vi "hydrolysis_reactor_run_parallel.vi"(10 "Spec files":path[](array[path]), 11 "instances":i32) -> (2 "paths out":path[](array[path]))   [LabVIEW 2019]
uses:
  <vilib>/Utility/sysdir.llb/System Directory Type.ctl
  lib/libSimulationControl/libSimulationControl.lvlib
panel:
  # "*******************************************************************\nBiogas Plant Control\n\nAuthor: Paul Zügel\nGCSC-Frankfurt am Main 2020\n\n*******************************************************************"
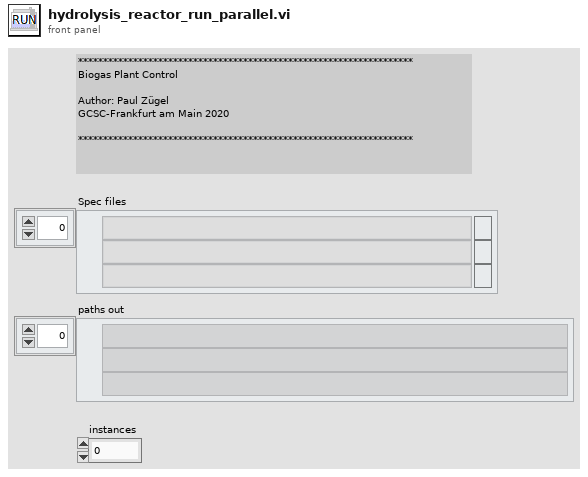
[diagram p1: front panel]
types:
  T1 = typedef "System Directory Type.ctl" = i32
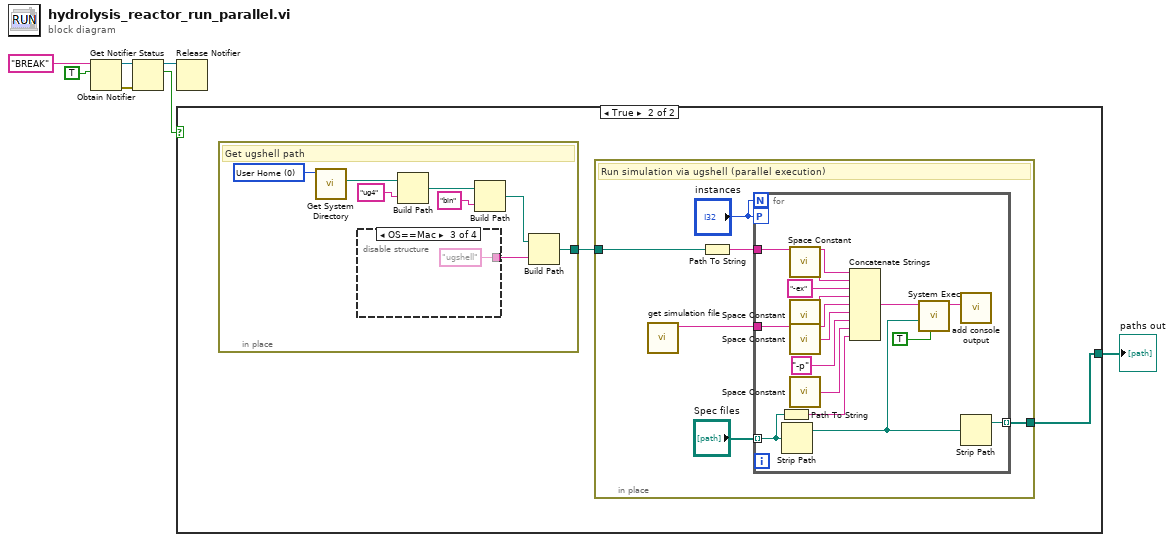
[diagram p0: block diagram]
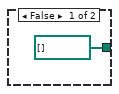
[diagram p2: hidden frame]
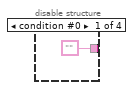
[diagram p3: hidden frame]
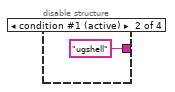
[diagram p4: hidden frame]
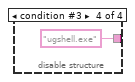
[diagram p5: hidden frame]
diagram:
  n1 = Obtain Notifier(name (unnamed)="BREAK", notification data type=TRUE) -> (notifier out=w5:refnum<notifier>, error out=w4:errorcluster)  [unwired: 2 in, 1 out]
  n2 = Get Notifier Status(notifier=w5, error in (no error)=w4) -> (notifier out=w1:refnum<notifier>, current notification=w3:bool)  [unwired: 3 out]
  n3 = Release Notifier(notifier=w1) -> ()  [unwired: 2 in, 3 out]
  n4 = case shown="True" w3 {
    tunnel: [path[] [] ("Spec files") w10] -> w2
    frame False {
    }
    frame True {
      # "Define current paths"
      # "True only on first Iteration (current_time = starttime)\nWe get all names of output Files from the outputFiles.lua and copy them from tmp to the working directory."
      n5 = in-place {
        in-place-border: [w11] -> w9
        w12 = T1 0 items=["User Home"=0, "User Desktop"=1, "User Documents"=2, "User Application Data"=3, "User Preferences"=4, "User Temporary"=5, "Public Documents"=6, "Public Application Data"=7, "Public Preferences"=8, "Public Cache"=13, "System Core Libraries"=9, "System Installed Libraries"=10, "Application Files"=11, "Boot Volume Root"=12] ("system directory type")
        # "Get ugshell path"
        n6 = call <vilib>:"Get System Directory.vi"("system directory type"=w12) -> ("system directory"=w15:path)  [unwired: 10 in]
        n7 = disable-structure shown="OS==Mac" {
          disable-tunnel: ["" "ugshell" ("name or relative path") "ugshell" ("name or relative path") "ugshell.exe" ("name or relative path")] -> w18
          frame condition #0 {
          }
          frame condition #1 (active) {
          }
          frame condition #2 {
          }
          frame condition #3 {
          }
        }
        n8 = Build Path(base path=w15, name or relative path="ug4") -> (appended path=w16:path)
        n9 = Build Path(base path=w16, name or relative path="bin") -> (appended path=w17:path)
        n10 = Build Path(base path=w17, name or relative path=w18) -> (appended path=w11:path)
      }
      n11 = in-place {
        in-place-border: [w26] -> w10
        in-place-border: w9 -> [w24]
        # "Run simulation via ugshell (parallel execution)"
        n12 = call "get simulation file.vi"() -> ("function return"=w28:string)  [unwired: 10 in, 1 out]
        n13 = Path To String(path=w24) -> (string=w23:string)
        n14 = for {
          N: "instances" -> [_]
          tunnel: w28 -> [w35]
          tunnel: w23 -> [w33]
          tunnel: "Spec files" -> [w31] mode=indexing
          workers-P: "instances" -> [_]
          tunnel: [w29] -> w26 mode=indexing
          n15 = Path To String(path=w31) -> (string=w32:string)
          n16 = Strip Path(path=w31) -> (stripped path=w30:path)  [unwired: 1 out]
          n17 = call <vilib>:"Space Constant.vi"() -> ("String"=w38:string)
          n18 = call <vilib>:"Space Constant.vi"() -> ("String"=w39:string)
          n19 = call <vilib>:"Space Constant.vi"() -> ("String"=w40:string)
          n20 = call <vilib>:"Space Constant.vi"() -> ("String"=w42:string)
          n21 = Concatenate Strings(w33, w38, "-ex" ("command line"), w39, w35, w40, "-p" ("command line"), w42, w32) -> (w41:string)
          n22 = call <vilib>:"System Exec.vi"("run minimized? (F)"=TRUE, "working directory"=w30, "command line"=w41) -> ("standard output"=w43:string)  [unwired: 5 in, 3 out]
          n23 = call "add console output.vi"("add_to_console"=w43) -> ()  [unwired: 11 in]
          n24 = Strip Path(path=w30) -> (stripped path=w29:path)  [unwired: 1 out]
        }
      }
    }
  }
  "paths out" <- w2
